vi "APP Open Stand Alone Interface.vi"(2 "Menubar":refnum<k9>, 11 "Error In (no error)":errorcluster) -> (3 "Local APP Setup Out":T1, 4 "Stand Alone":bool, 15 "Error Out":errorcluster)   [LabVIEW 2011]
uses:
  Type Defs/APP Application Setup Cluster.ctl
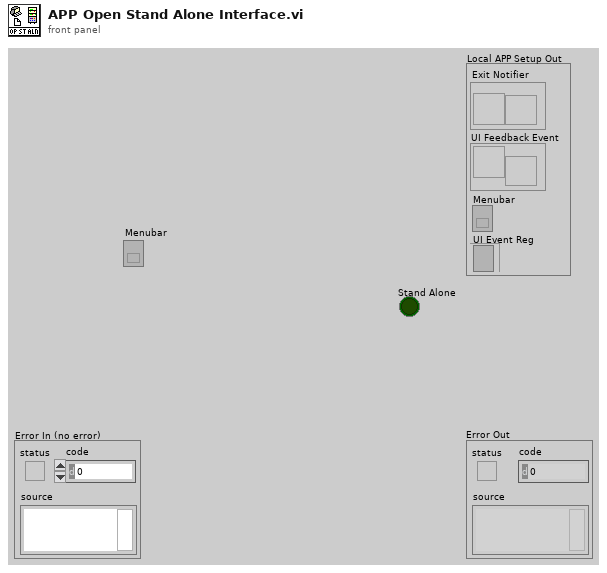
[diagram p1: front panel]
types:
  T1 = typedef "APP Application Setup Cluster.ctl" = cluster{"Menubar":refnum<k9>, "Exit Notifier":refnum<notifier>, "UI Feedback Event":refnum<user-event>, "UI Event Reg":refnum<event-registration>}
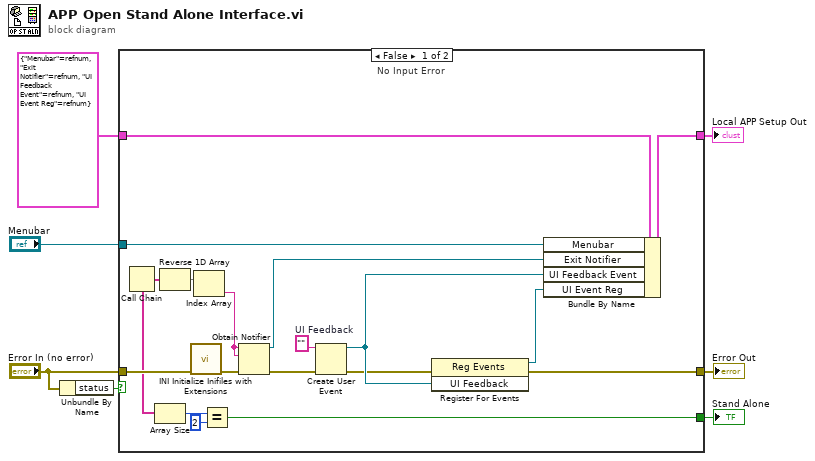
[diagram p0: block diagram]
diagram:
  n1 = Unbundle By Name("Error In (no error)") -> ("status"=w1:bool)
  n2 = case shown="False" w1 {
    tunnel: [w13 w27] -> w6
    tunnel: "Error In (no error)" -> [w18 w27]
    tunnel: [w25 w26] -> w4
    tunnel: "Menubar" -> [w23 _]
    tunnel: T1 {"Menubar"=refnum, "Exit Notifier"=refnum, "UI Feedback Event"=refnum, "UI Event Reg"=refnum} ("Local APP Setup Out") -> [w19 w26]
    tunnel: [w9 _] -> w5
    frame False {
      w20 = ""  # UI Feedback
      # "No Input Error"
      n3 = Call Chain() -> (call chain=w11:string[])
      n4 = Array Size(array=w11) -> (size(s)=w10:i32)
      n5 = Reverse 1D Array(array=w11) -> (reversed array=w22:string[])
      n6 = call "INI Initialize Inifiles with Extensions.vi"("Error In (no error)"=w18) -> ("Error Out"=w17:errorcluster)  [unwired: 13 in, 1 out]
      n7 = Index Array(array=w22) -> (element=w14:string)  [unwired: 1 in]
      n8 = Equal?(x=w10, y=2) -> (x = y?=w9:bool)
      n9 = Obtain Notifier(name (unnamed)=w14, notification data type=w14, error in (no error)=w17) -> (notifier out=w24:refnum<notifier>, error out=w21:errorcluster)  [unwired: 1 in, 1 out]
      n10 = Create User Event(user event datatype=w20, error in=w21) -> (user event=w16:refnum<user-event>, error out=w8:errorcluster)
      n11 = register-events(error in=w8, w16) -> (reference out=w15:refnum<event-registration>, error out=w13:errorcluster)  [unwired: 1 in]
      n12 = Bundle By Name(cluster=w19, "Menubar"=w23, "Exit Notifier"=w24, "UI Feedback Event"=w16, "UI Event Reg"=w15) -> (w25:T1)
    }
    frame True {
      # "Input Error"
    }
  }
  "Error Out" <- w6
  "Stand Alone" <- w5
  "Local APP Setup Out" <- w4
